vi "TestChart.vi"() -> ()   [LabVIEW 2014]
panel:
  out "ChartOut":picture
  in  "stop":bool
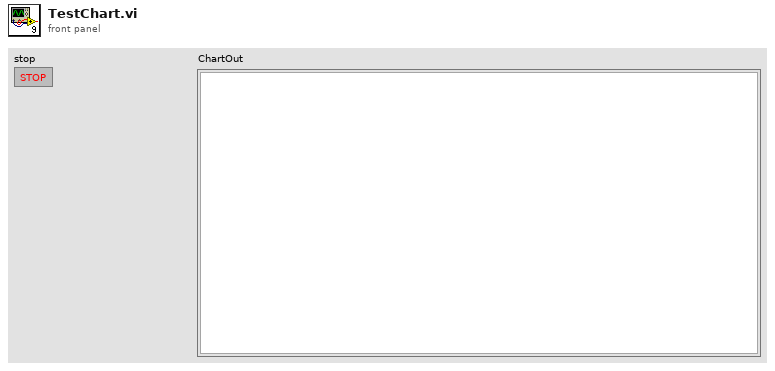
[diagram p1: front panel]
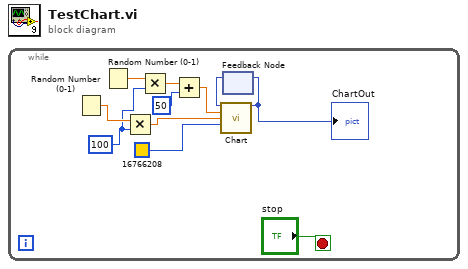
[diagram p0: block diagram]
diagram:
  n1 = while {
    stop <- "stop" stop-if-true
    w4 = 100
    n2 = Random Number (0-1)() -> (number: 0 to 1=w10:dbl)
    n3 = Random Number (0-1)() -> (number: 0 to 1=w5:dbl)
    n4 = Multiply(x=w10, y=w4) -> (x*y=w9:dbl)
    n5 = Multiply(x=w5, y=w4) -> (x*y=w3:dbl)
    n6 = Add(x=w3, y=50) -> (x+y=w1:dbl)
    n7 = feedback #1() -> (w7:picture)  [unwired: 1 in]
    n8 = call "Chart.vi"("PictureIn"=w7, "x"=w1, "y"=w9, "colorRectangle"=u32 16766208) -> ("ChartOut"=w8:picture)  [unwired: 10 in, 1 out]
    "ChartOut" <- w8
    n9 = feedback-in #1(w8) -> ()
  }
